vi "CP_Undock_Position_Calc.vi"(8 "Offset":i32=25, 9 "subVI FP WinBounds In":T1, 10 "SubPanel Position":cluster{"Left":i32, "Top":i32}, 11 "Main FP WinBounds":T1) -> (1 "subVI FP Window Bounds Out":T1)   [LabVIEW 2009]
doc: "Part of the Dock/Undock demonstration of Sub Panels. Contributed by www.entzen.com.\n\nAAL 9/09"
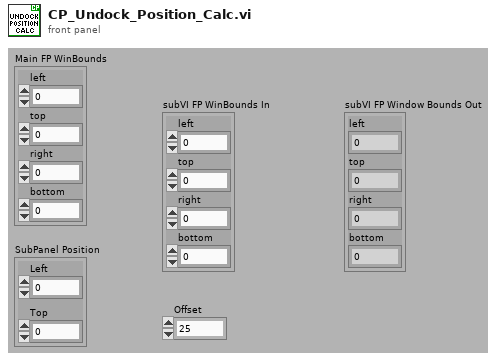
[diagram p1: front panel]
types:
  T1 = cluster{"left":i16, "top":i16, "right":i16, "bottom":i16}
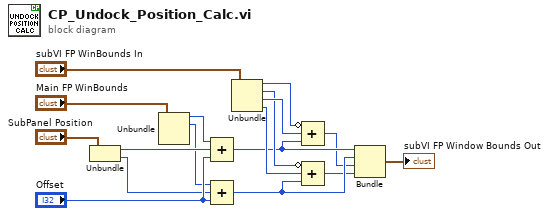
[diagram p0: block diagram]
diagram:
  n1 = Unbundle("SubPanel Position") -> ("Left"=w16:i32, "Top"=w13:i32)
  n2 = Unbundle("Main FP WinBounds") -> ("left"=w17:i16, "top"=w14:i16)  [unwired: 2 out]
  n3 = Compound Arithmetic op=ADD(w17, w16, "Offset") -> (w8:i32)
  n4 = Compound Arithmetic op=ADD(w14, w13, "Offset") -> (w7:i32)
  n5 = Unbundle("subVI FP WinBounds In") -> ("left"=w12:i16, "top"=w10:i16, "right"=w11:i16, "bottom"=w9:i16)
  n6 = Compound Arithmetic op=ADD(invert w12, w11, w8) -> (w6:i32)
  n7 = Compound Arithmetic op=ADD(invert w10, w9, w7) -> (w5:i32)
  n8 = Bundle(w8, w7, w6, w5) -> (→"subVI FP Window Bounds Out":cluster{i32, i32, i32, i32})  [unwired: 1 in]
